vi "MultirunBuilderForNamedLocations.vi"() -> ()   [LabVIEW 2015]
uses:
  Anemometry Sub Vis/Controls/MeasureInLoop.ctl
  Anemometry Sub Vis/Controls/MeasurementLocation.ctl
  Anemometry Sub Vis/Gen Trav/Spacing.ctl
  Anemometry Sub Vis/Controls/Multi_run_mode.ctl
  Anemometry Sub Vis/File/Setup_Filetype.ctl
  Anemometry Sub Vis/Globals/Meas_global.vi
panel:
  in  "RowTemplate":T3 {"Carrier_2 Q (l/min)" format="%#.2f"; "Row Duration (mins)" format="%#.1f"; "Row No" min=0; "Trace Gas Concentration (%)" min=0.0 format="%#_4f"; "Carrier_1 Q (l/min)" format="%#.2f"; "Tunnel Speed" format="%#.2f"; "Start X" format="%#.2f"; "Start Y" format="%#.2f"; "Start Z" format="%#.2f"; "End X" format="%#.2f"; "End Y" format="%#.2f"; "End Z" format="%#.2f"; "Averaging time (min)" min=0.0 format="%#.2f"}
  in  "Tab Control":T4(tab)
  in  "Azimuths":dbl[](array[numeric])=[0.0, 20.0, 40.0, 60.0, 80.0, 100.0, 120.0, 140.0, 160.0, 180.0, 200.0, 220.0, 240.0, 260.0, 280.0, 300.0, 320.0, 340.0]
  in  "ZsAboveRoof":sgl[](array[numeric])=[16.8, 25.4, 33.9]
  in  "Locations":T5[](array[typedef]) caption="X                          Y                    RoofZ                        Name"
  in  "Local Calcheck Location":cluster{"X":dbl, "Y":dbl, "Z":dbl} caption="Global Calc"
  in  "Global Calcheck Location":cluster{"X":dbl, "Y":dbl, "Z":dbl} caption="Global Calc"
  in  "Tunnel Warmup (min)":dbl=20.0
  in  "Velocity (m/s)":dbl=9.0
  in  "Measure (seconds)":dbl=60.0
  in  "Setup:":string(combo)="Current_Setup.xls"
  out "Task":T6=enum."Initialise"
  in  "Stop Button":bool
  # "X           Y            Z"
  # "Start"
  # "End"
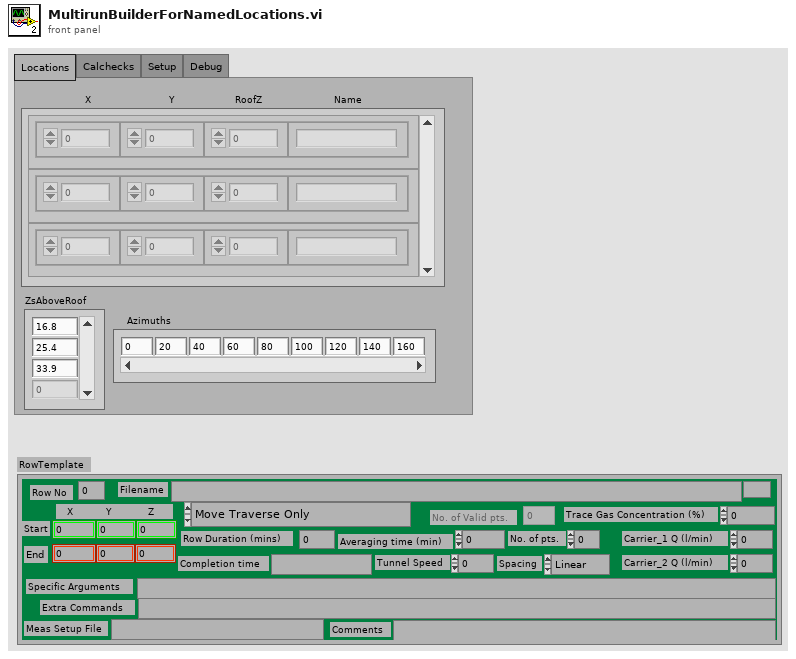
[diagram p1: front panel]
types:
  T1 = typedef "Spacing.ctl" = enum16{"Linear", "Log", "Gauss", "Specified", "N/A"}
  T2 = typedef "Multi_run_mode.ctl" = enum16{"Move Traverse Only", "Set Tunnel Speed Only", "Set Source Only", "Set Measurement Conditions", "Single Measurement", "Vertical Profile", "Lateral Profile", "Longitudinal Profile", "Explore Volume", "Multi-Axis Profile", "Auto Calibrate", "Meas Fast FID Bkgnd", "Check Beam Power", "Scanning Valve Measurement", "Run VI Named:", "Set ADAM Ch", "Wait (minutes)", "Send Message", "Synchronize With:", "Fall Back to this Row", "Turn Off Row Repeating", "Blank Row", "Traverse 3D Volume"}
  T3 = cluster{"Start X":sgl, "Start Y":sgl, "Start Z":sgl, "End X":sgl, "End Y":sgl, "End Z":sgl, "No. of pts.":i32, "Spacing":T1, "Filename":path, "Tunnel Speed":dbl, "Averaging time (min)":dbl, "Extra Commands":string, "Carrier_1 Q (l/min)":dbl, "Carrier_2 Q (l/min)":dbl, "Trace Gas Concentration (%)":dbl, "Specific Arguments":string, "Comments":string, "Row No":i32, "Row Type Selector":T2, "Completion time":string, "Row Duration (mins)":dbl, "No. of Valid pts.":i32, "Meas Setup File":string}
  T4 = enum32{"Locations", "Calchecks", "Setup", "Debug"}
  T5 = typedef "MeasurementLocation.ctl" = cluster{"X":sgl, "Y":sgl, "LocalZ0":sgl, "Name":string}
  T6 = typedef "MeasureInLoop.ctl" = enum16{"RunHub", "Initialise", "Take Measurement", "Start Waiting", "End"}
  T7 = typedef "Setup_Filetype.ctl" = enum16{"Measurement Setups", "Calibration Setups", "General", "Results File Plotter Setups", "Speed Calib Tweaks"}
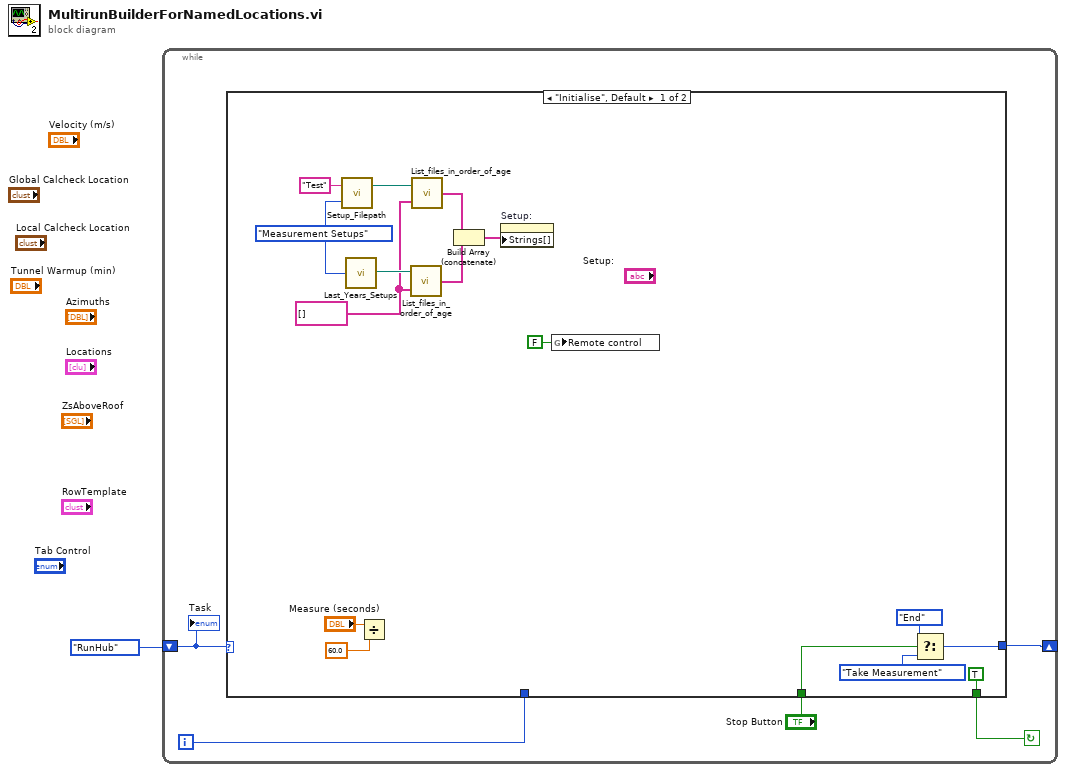
[diagram p0: block diagram]
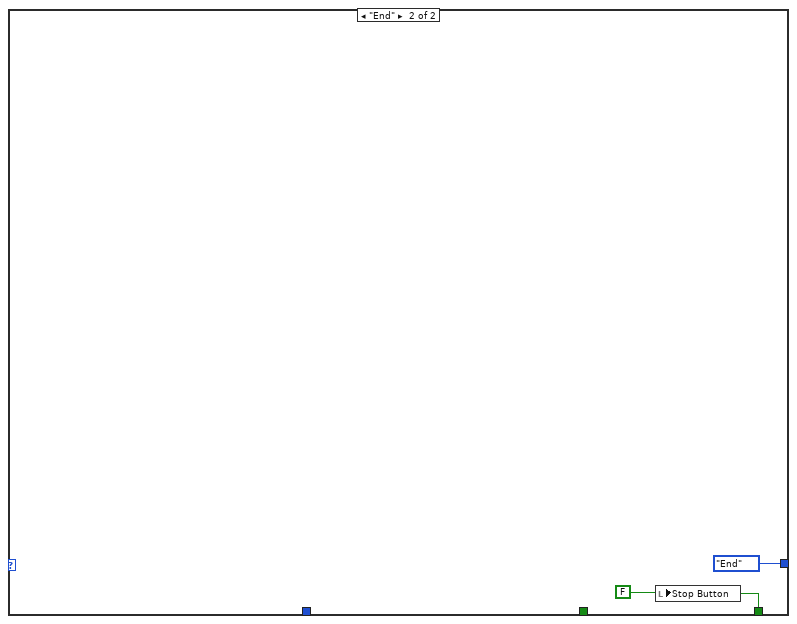
[diagram p2: hidden frame]
diagram:
  n1 = while {
    shift-right: [w5] -> _
    shift-left: MeasureInLoop."RunHub" ("Task") -> [w3]
    i -> [w6]
    stop <- w4 continue-if-true
    n2 = case shown="\"Initialise\", Default" w3 {
      tunnel: w6 -> [_ _]
      tunnel: [w9 MeasureInLoop."End" ("Task")] -> w5
      tunnel: [TRUE ("Stop Button") w23] -> w4
      tunnel: "Stop Button" -> [w7 _]
      frame "Initialise", Default {
        w19 = Setup_Filetype."Measurement Setups" ("Setup File Type")
        w14 = string[] [] ("file names")
        n3 = call "Setup_Filepath.vi"("Setup File Type"=w19, "Filename in"="Test") -> ("Directory"=w18:path)  [unwired: 1 out]
        n4 = call "Last_Years_Setups.vi"("Setup File Type"=w19) -> ("Directory"=w20:path)
        n5 = Divide(x="Measure (seconds)", y=60.0 ("x")) -> ()  [unwired: 1 out]
        n6 = call "List_files_in_order_of_age.vi"("Files to Hide"=w14, "Folder"=w20) -> ("file names"=w16:string[])
        n7 = call "List_files_in_order_of_age.vi"("Files to Hide"=w14, "Folder"=w18) -> ("file names"=w17:string[])
        n8 = Build Array (concatenate)(w17, w16) -> (w13:string[])
        n9 = property on="Setup:" class="CmbBox"("Strings[]"=w13) -> ()  [unwired: 2 in, 2 out]
        n10 = global write "Meas_global.vi" "Remote control"(FALSE ("Remote control")) -> ()
        n11 = Select(t=MeasureInLoop."End" ("Task"), s=w7, f=MeasureInLoop."Take Measurement" ("Task")) -> (s? t:f=w9:T6)
      }
      frame "End" {
        w23 = FALSE ("Stop Button")
        n12 = local write "Stop Button"(w23) -> ()
      }
    }
    "Task" <- w3
  }
